vi "Get All Properties.vi"(8 "error in":errorcluster) -> (0 "error out":errorcluster, 3 "Properties[]":T1(array[cluster]))   [LabVIEW 2023]
panel:
  out "Classes processed":i32
  out "Class processing":string
  out "Property Ct":i32
  out "exe time (ms)":u32
  # "Original time was ca 5 min, improved class sorting and made sure we don't get properties for a class more than once:\n\n2504 props, 231 processed, 65s\n2504, 295 processed, 81s\n2504, 230 processed, 79s.\n\nLooks like sorting classes isn't needed\n\nNext round of improvement, put helper VI refs in shift registers so we don't get class and proeprty node rein a loop\n\n2504, props, 25s. Wow!!!\n\nLV2023 9-24\n2519 properties in 9.5s"
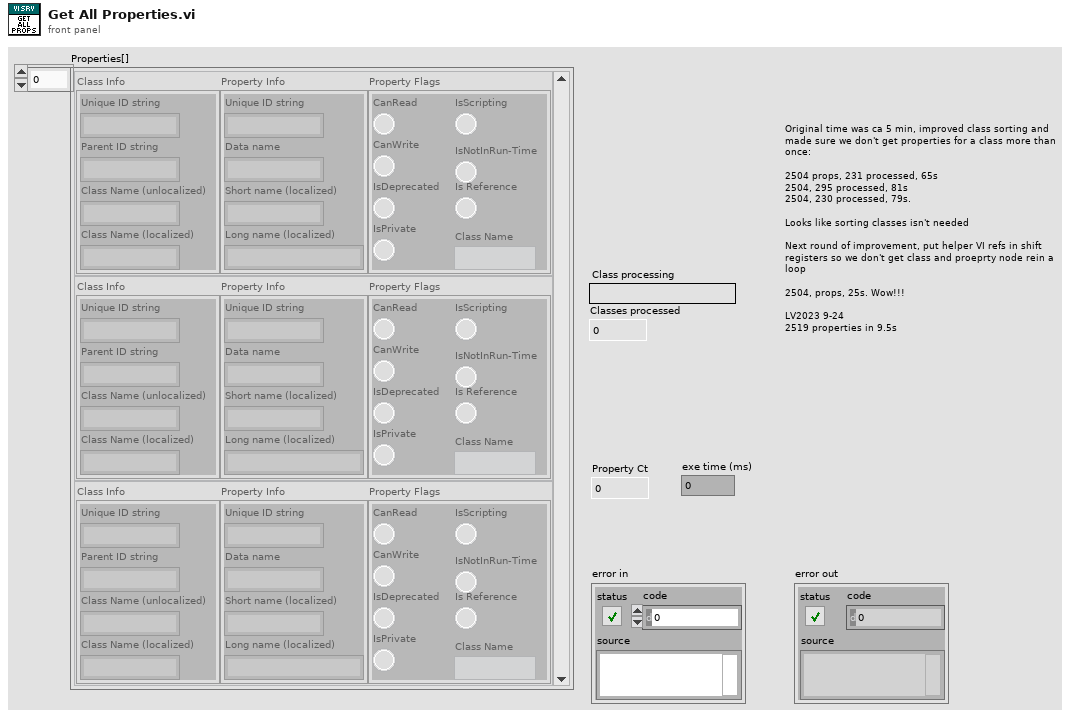
[diagram p1: front panel]
types:
  T1 = cluster{"Class Info":cluster{"Unique ID string":string, "Parent ID string":string, "Class Name (unlocalized)":string, "Class Name (localized)":string}, "Property Info":cluster{"Unique ID string":string, "Data name":string, "Short name (localized)":string, "Long name (localized)":string}, "Property Flags":cluster{"CanRead":bool, "CanWrite":bool, "IsDeprecated":bool, "IsPrivate":bool, "IsScripting":bool, "IsNotInRun-Time":bool, "Is Reference":bool, "Class Name":string}}[]
  T2 = cluster{"Unique ID string":string, "Parent ID string":string, "Class Name (unlocalized)":string, "Class Name (localized)":string}[]
  T3 = cluster{"Done":refnum<user-event>, "Msg 1":refnum<user-event>, "Msg 2":refnum<user-event>, "Prog Max":refnum<user-event>, "Prog Ct":refnum<user-event>}
  T4 = cluster{"Class Name":string, "Property Info":cluster{"Unique ID string":string, "Data name":string, "Short name (localized)":string, "Long name (localized)":string}}[]
  T5 = cluster{"Unique ID string":string, "Data name":string, "Short name (localized)":string, "Long name (localized)":string}
  T6 = cluster{"CanRead":bool, "CanWrite":bool, "IsDeprecated":bool, "IsPrivate":bool, "IsScripting":bool, "IsNotInRun-Time":bool, "Is Reference":bool, "Class Name":string}
  T7 = cluster{"Property/Method Info":cluster{"Unique ID string":string, "Parent ID string":string, "Class Name (unlocalized)":string, "Class Name (localized)":string}, "Property Info":cluster{"Unique ID string":string, "Data name":string, "Short name (localized)":string, "Long name (localized)":string}, "Property Flags":cluster{"CanRead":bool, "CanWrite":bool, "IsDeprecated":bool, "IsPrivate":bool, "IsScripting":bool, "IsNotInRun-Time":bool, "Is Reference":bool, "Class Name":string}}
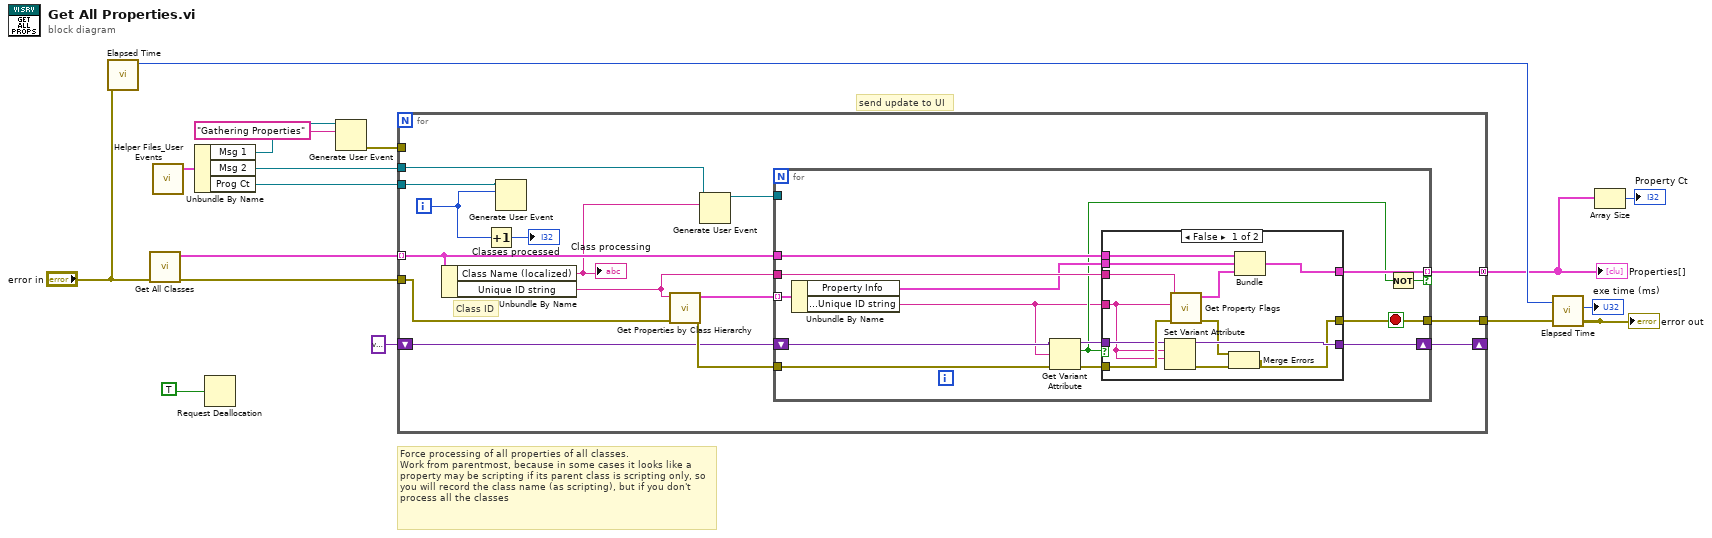
[diagram p0: block diagram]
diagram:
  # "send update to UI"
  # "Force processing of all properties of all classes.\nWork from parentmost, because in some cases it looks like a property may be scripting if its parent class is scripting only, so you will record the class name (as scripting), but if you don't process all the classes"
  n1 = call "Elapsed Time.vi"("error in"="error in") -> ("millisecond timer value"=w14:u32)  [unwired: 6 in, 4 out]
  n2 = call "Get All Classes.vi"("error in (no error)"="error in") -> ("error out"=w16:errorcluster, "VI Server Classes[]"=w11:T2)  [unwired: 9 in]
  n3 = call "Helper Files_User Events.vi"() -> ("Init Dialog UEs"=w7:T3)  [unwired: 11 in]
  n4 = Unbundle By Name(w7) -> ("Msg 1"=w4:refnum<user-event>, "Msg 2"=w6:refnum<user-event>, "Prog Ct"=w5:refnum<user-event>)
  n5 = Request Deallocation(TRUE ("flag")) -> ()
  n6 = Generate User Event(user event=w4, event data cluster="Gathering Properties" ("event data")) -> (error out=w2:errorcluster)  [unwired: 2 in, 1 out]
  n7 = for {
    tunnel: w16 -> [w31]
    tunnel: [w23] -> w8
    shift-right: [w28] -> _
    shift-left: variant -> [w27]
    tunnel: [w25] -> w9 mode=concatenating
    tunnel: w11 -> [w22] mode=indexing
    tunnel: w6 -> [w21]
    tunnel: w5 -> [w19]
    tunnel: w2 -> [_]
    i -> [w18]
    # "Class ID"
    n8 = Unbundle By Name(w22) -> ("Class Name (localized)"=w17:string, "Unique ID string"=w26:string)
    "Class processing" <- w17
    n9 = Increment(x=w18) -> (x+1=→"Classes processed":i32)
    n10 = Generate User Event(user event=w19, event data cluster=w18) -> ()  [unwired: 2 in, 2 out]
    n11 = call "Get Properties by Class Hierarchy.vi"("error in (no error)"=w31, "Class ID"=w26) -> ("error out"=w30:errorcluster, "Properties by Class Hierarchy"=w29:T4)  [unwired: 7 in, 1 out]
    n12 = Generate User Event(user event=w21, event data cluster=w17) -> (user event out=w20:refnum<user-event>)  [unwired: 2 in, 1 out]
    n13 = for {
      tunnel: w29 -> [w35] mode=indexing
      tunnel: w22 -> [w37]
      tunnel: w30 -> [w44]
      tunnel: [w45] -> w23
      shift-right: [w42] -> w28
      shift-left: w27 -> [w41]
      tunnel: w26 -> [w39]
      tunnel: [w38] -> w25 mode=indexing if=w33
      tunnel: w20 -> [_]
      stop <- w45 stop-if-true
      n14 = Unbundle By Name(w35) -> ("Property Info"=w36:T5, "Property Info.Unique ID string"=w32:string)
      n15 = Get Variant Attribute(Variant=w41, name=w32, error in=w44) -> (duplicate Variant=w40:variant, found=w34:bool, error out=w43:errorcluster)  [unwired: 1 in, 1 out]
      n16 = case shown="False" w34 {
        tunnel: w39 -> [w46 _]
        tunnel: w37 -> [w57 _]
        tunnel: [w47 w59] -> w45
        tunnel: w36 -> [w56 _]
        tunnel: w43 -> [w55 w59]
        tunnel: w32 -> [w50 _]
        tunnel: [w53 w58] -> w42
        tunnel: w40 -> [w52 w58]
        tunnel: [w51 _] -> w38
        frame False {
          n17 = Set Variant Attribute(Variant=w52, name=w50, value=w50) -> (Variant out=w53:variant, error out=w49:errorcluster)  [unwired: 1 in, 1 out]
          n18 = call "Get Property Flags.vi"("error in (no error)"=w55, "Property ID"=w50, "Class ID"=w46) -> ("error out"=w48:errorcluster, "Property Flags"=w54:T6)  [unwired: 7 in]
          n19 = Merge Errors(w48, w49) -> (w47:errorcluster)
          n20 = Bundle("Property/Method Info"=w57, "Property Info"=w56, "Property Flags"=w54) -> (w51:T7)  [unwired: 1 in]
        }
        frame True {
        }
      }
      n21 = Not(x=w34) -> (.not. x?=w33:bool)
    }
  }
  "Properties[]" <- w9
  "error out" <- w8
  n22 = call "Elapsed Time.vi"("error in"=w8, "past time"=w14) -> ("elapsed time (ms)"=→"exe time (ms)":u32)  [unwired: 5 in, 4 out]
  n23 = Array Size(array=w9) -> (size(s)=→"Property Ct":i32)
